vi "Signal Monitor.vi"() -> ()   [LabVIEW 2010]
uses:
  DAQ configuration/port to indices.vi
  DataServer/command.ctl
  DataServer/command cluster.ctl
  support/method.ctl
  DAQ configuration/channel identifier.ctl
  DAQ configuration/Sensor array.ctl
panel:
  in  "Sensor Array":T1
  out "digital display":sgl[](array[numeric]) format="%.4e"
  out "scans acquired":u32
  in  "Chart":bool
  out "seconds":u32
  out "backlog":u32
  out "data server address":string="calcium"
  in  "Data Servers":string[](array[string])=["dataserver.cee.cornell.edu", "calcium.cee.cornell.edu"]
  in  "method":T3={"sampling interval"=0.1, "samples to average"=1, "data interval"=0.0, "stream data"=FALSE, "file path"=refnum, "command"={"command"=enum."Idle", "start time (ms)"=0, "Channel Indices"=[], "Scans per Sample"=1}} {"command"."Scans per Sample" min=1; "data interval" format="%.2f"; "samples to average" min=1 step=1; "sampling interval" format="%.2f"}
  in  "Data log status":bool
  in  "Enable Logging data":bool
  in  "colors":u32[](array[colorbox])=[16711680, 16770090, 6487897, 16777215, 16753241, 16738047, 52479, 2556143, 16711680, 16770090, 7470980, 16777215, 16753241, 16738047, 52479, 2556143]
  out "error":errorcluster
  out "chart":sgl[][](graph)
  in  "port":u16=6341
  out "connection ID":refnum<k5>
  out "quit":bool=TRUE
  in  "State":T6
  in  "Stop":bool
  in  "Log Data":bool
  out "logging data to file:":path=path "C:/WINNT/Profiles/mlws/Desktop/50Hzjunk"
  # "current value"
  # "channel  name (units)"
  # "s"
  # "s"
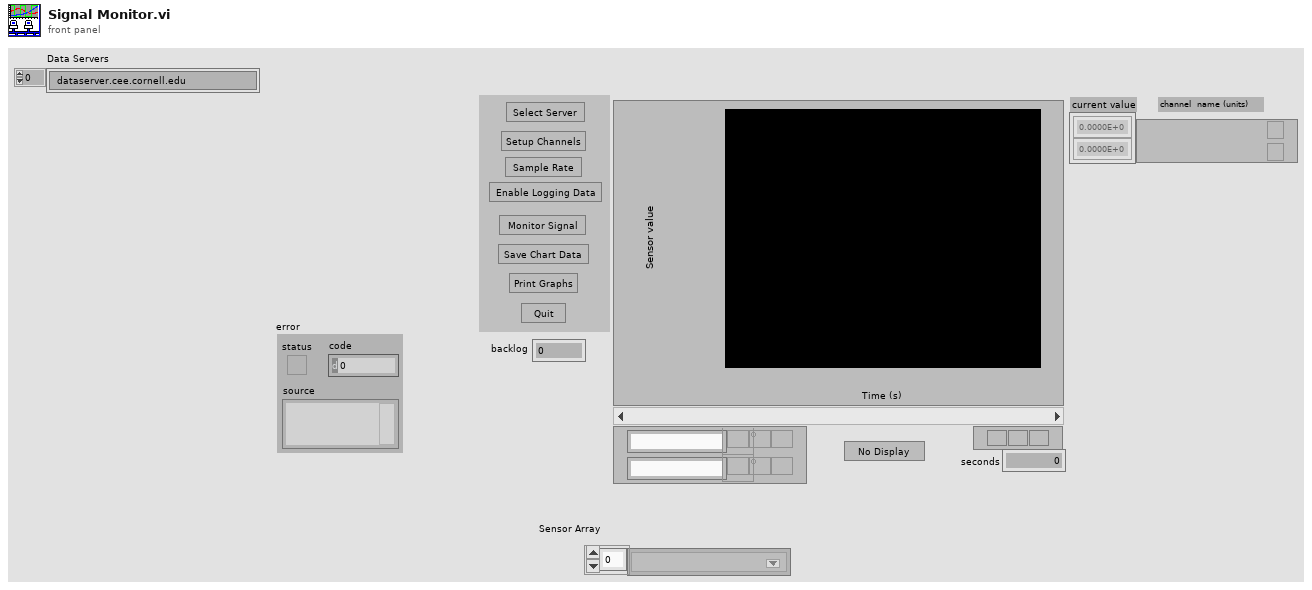
[diagram p1: front panel]
types:
  T1 = typedef "Sensor array.ctl" = T2[]
  T2 = typedef "channel identifier.ctl" = u16
  T3 = typedef "method.ctl" = cluster{"sampling interval":sgl, "samples to average":u32, "data interval":sgl, "stream data":bool, "file path":refnum<file>, "command":T4}
  T4 = typedef "command cluster.ctl" = cluster{"command":T5, "start time (ms)":u32, "Channel Indices":i32[], "Scans per Sample":i32}
  T5 = typedef "command.ctl" = enum16{"Idle", "Send Data", "Send 1 Scan", "Logoff"}
  T6 = cluster{"Quit":bool, "Select Server":bool, "Calibration":bool, "Set Rate":bool, "Monitor sample":bool, "Save data":bool, "Print graphs":bool}
  T7 = enum16{"Idle", "Send Data", "Send 1 Scan", "Logoff"}
  T8 = typedef "Sensor array.ctl" = T9[]
  T9 = typedef "sensor configuration.ctl" = cluster{"Port":T10, "calibration type":T11, "name":string}
  T10 = typedef "channel identifier.ctl" = cluster{"module":u8, "channel":u8}
  T11 = typedef "calibration type.ctl" = enum16{"None (raw voltage)", "From File", "Zero voltage", "Set calibrated output", "pH", "Dissolved Oxygen", "LVDT calibrator", "NF90 calibrator"}
  T12 = cluster{"X Scale Fit":u8, "Xo and delta X":cluster{"Xo":dbl, "delta X":dbl}, "X style":u8, "X Format & Precision":cluster{"X Format":u8, "X Precision":u8}, "X Range":cluster{"X Minimum":dbl, "X Maximum":dbl, "X Increment":dbl}, "X Flipped":bool, "X Mapping Mode":u8, "X Editable":bool}
  T13 = cluster{"Y Scale Fit":u8, "Yo and delta Y":cluster{"Yo":dbl, "delta Y":dbl}, "Y Style":u8, "Y Format & Precision":cluster{"Y Format":u8, "Y Precision":u8}, "Y Range":cluster{"Y Minimum":dbl, "Y Maximum":dbl, "Y Increment":dbl}, "Y Flipped":bool, "Y Mapping Mode":u8, "Y Editable":bool}
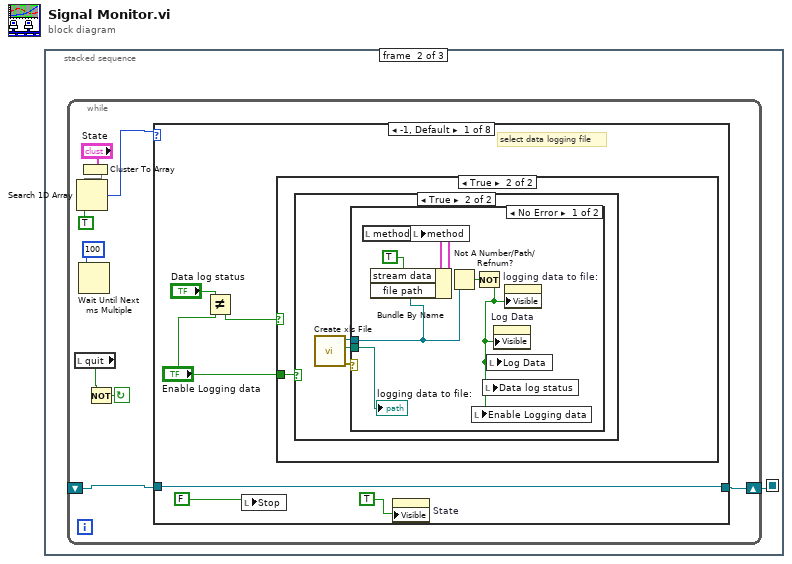
[diagram p0: block diagram]
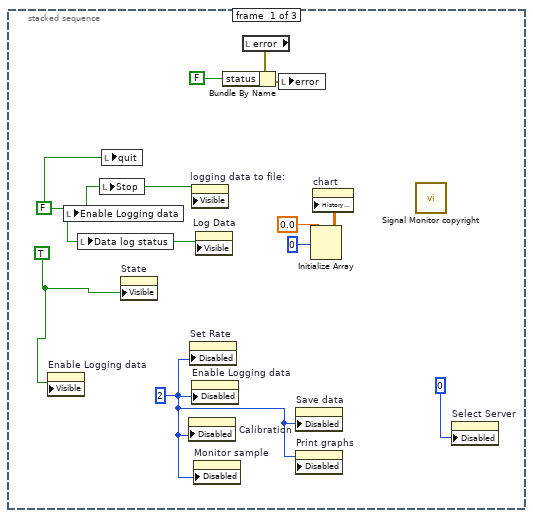
[diagram p2: hidden frame]
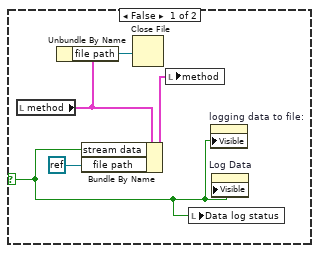
[diagram p4: hidden frame]
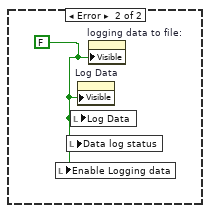
[diagram p5: hidden frame]
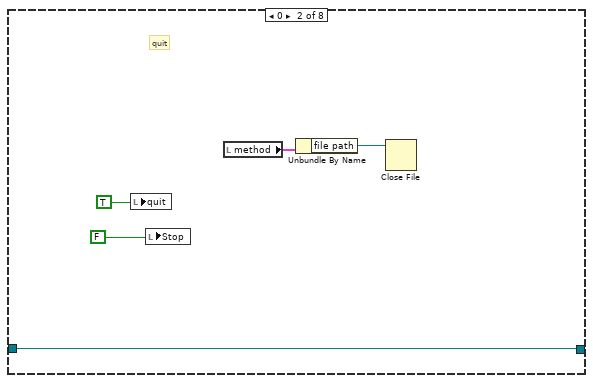
[diagram p6: hidden frame]
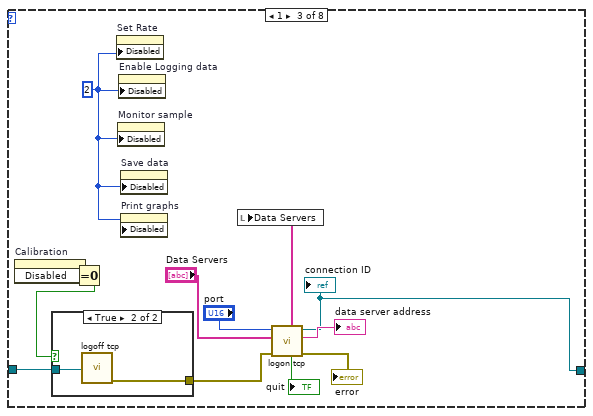
[diagram p7: hidden frame]
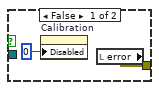
[diagram p8: hidden frame]
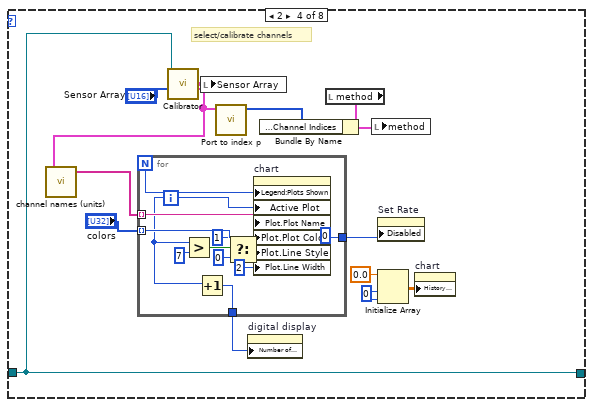
[diagram p9: hidden frame]
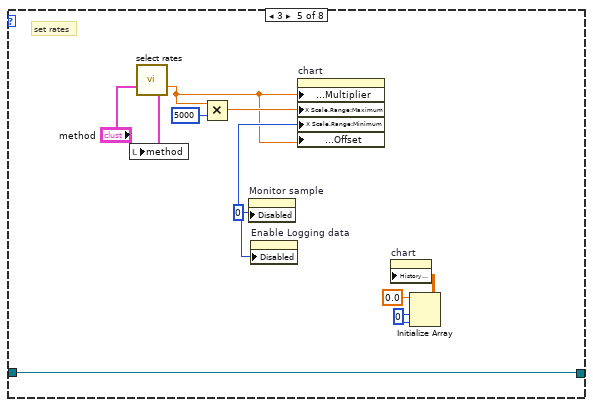
[diagram p10: hidden frame]
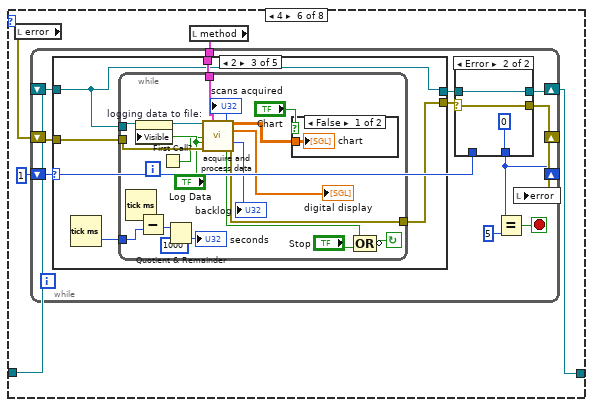
[diagram p11: hidden frame]
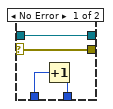
[diagram p12: hidden frame]
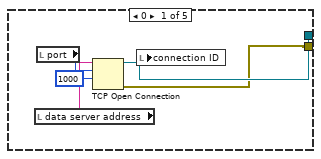
[diagram p13: hidden frame]
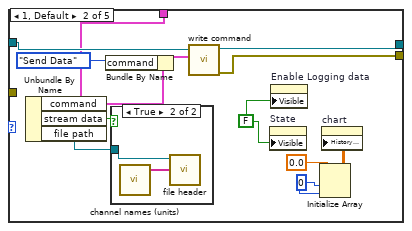
[diagram p14: hidden frame]
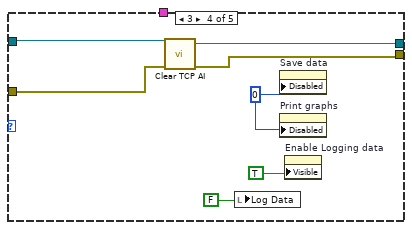
[diagram p17: hidden frame]
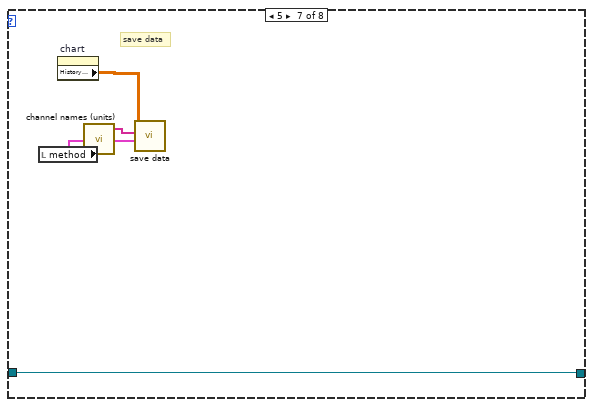
[diagram p19: hidden frame]
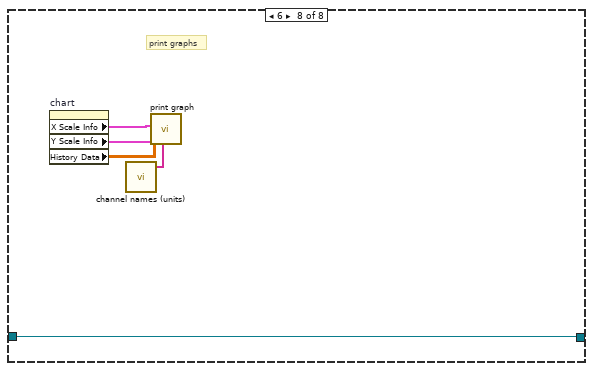
[diagram p20: hidden frame]
diagram:
  n1 = stacked-sequence {
    seq-local: [_ w11 _] -> [_ _ w186]
    frame #0 {
      w6 = TRUE
      w5 = 2
      w8 = 0
      w7 = FALSE
      n2 = property on="Enable Logging data" class="Bool (strict)"("Visible"=w6) -> ()  [unwired: 2 in, 2 out]
      n3 = local write "Enable Logging data"(w7) -> ()
      n4 = local write "Data log status"(w7) -> ()
      n5 = local write "Stop"(w7) -> ()
      n6 = local write "quit"(w7) -> ()
      n7 = property on="State" class="Clust"("Visible"=w6) -> ()  [unwired: 2 in, 2 out]
      n8 = property on="Calibration" class="Bool"("Disabled"=w5) -> ()  [unwired: 2 in, 2 out]
      n9 = property on="Set Rate" class="Bool"("Disabled"=w5) -> ()  [unwired: 2 in, 2 out]
      n10 = property on="logging data to file:" class="Path"("Visible"=w7) -> ()  [unwired: 2 in, 2 out]
      n11 = property on="Enable Logging data" class="Bool (strict)"("Disabled"=w5) -> ()  [unwired: 2 in, 2 out]
      n12 = property on="Monitor sample" class="Bool"("Disabled"=w5) -> ()  [unwired: 2 in, 2 out]
      n13 = property on="Log Data" class="Bool (strict)"("Visible"=w7) -> ()  [unwired: 2 in, 2 out]
      n14 = local read "error"() -> (w3:errorcluster)
      n15 = Bundle By Name(cluster=w3, "status"=FALSE ("Bundle Element")) -> (w2:errorcluster)
      n16 = local write "error"(w2) -> ()
      n17 = property on="Save data" class="Bool"("Disabled"=w5) -> ()  [unwired: 2 in, 2 out]
      n18 = property on="Print graphs" class="Bool"("Disabled"=w5) -> ()  [unwired: 2 in, 2 out]
      n19 = Initialize Array(sgl 0.0, w8, w8) -> (w9:sgl[][])
      n20 = property on="chart" class="WFChart (strict)"("History Data"=w9) -> ()  [unwired: 2 in, 2 out]
      n21 = call "Signal Monitor copyright"() -> ()  [unwired: 8 in]
      n22 = property on="Select Server" class="Bool"("Disabled"=u8 0 ("Write Attribute")) -> ()  [unwired: 2 in, 2 out]
    }
    frame #1 {
      n23 = while {
        shift-left: _ -> [w13]
        shift-right: [w12] -> w11
        stop <- w19 continue-if-true
        n24 = local read "quit"() -> (w20:bool)
        n25 = Wait Until Next ms Multiple(millisecond multiple=100) -> ()  [unwired: 1 out]
        n26 = Cluster To Array(cluster="State") -> (array=w17:bool[])
        n27 = Search 1D Array(1D array=w17, element=TRUE) -> (index of element=w16:i32)  [unwired: 1 in]
        n28 = Not(x=w20) -> (.not. x?=w19:bool)
        n29 = case shown="-1, Default" w16 {
          tunnel: w13 -> [w21 w46 w54 w77 w94 w103 w177 w181]
          tunnel: [w21 w46 w56 w77 w94 w102 w177 w181] -> w12
          frame -1, Default {
            # "select data logging file"
            n30 = Not Equal?(x="Data log status", y="Enable Logging data") -> (x != y?=w22:bool)
            n31 = local write "Stop"(FALSE) -> ()
            n32 = case shown="True" w22 {
              tunnel: "Enable Logging data" -> [_ w27]
              frame False {
              }
              frame True {
                n33 = case shown="True" w27 {
                  selector: w27 -> [w30 _]
                  frame False {
                    n34 = local read "method"() -> (w29:T3)
                    n35 = Unbundle By Name(w29) -> ("file path"=w28:refnum<file>)
                    n36 = Bundle By Name(cluster=w29, "stream data"=w30, "file path"=refnum<k0> refnum) -> (w32:T3)
                    n37 = Close File(refnum=w28) -> ()  [unwired: 1 in, 2 out]
                    n38 = local write "method"(w32) -> ()
                    n39 = local write "Data log status"(w30) -> ()
                    n40 = property on="logging data to file:" class="Path"("Visible"=w30) -> ()  [unwired: 2 in, 2 out]
                    n41 = property on="Log Data" class="Bool (strict)"("Visible"=w30) -> ()  [unwired: 2 in, 2 out]
                  }
                  frame True {
                    n42 = call "Create xls File.vi"() -> ("error out"=w34:errorcluster, "path"=w33:path, "refnum"=w35:refnum<file>)  [unwired: 4 in, 1 out]
                    n43 = case shown="No Error" w34 {
                      tunnel: w35 -> [w36 _]
                      tunnel: w33 -> [w37 _]
                      frame No Error {
                        n44 = local read "method"() -> (w40:T3)
                        n45 = Bundle By Name(cluster=w40, "stream data"=TRUE, "file path"=w36) -> (w41:T3)
                        n46 = local write "method"(w41) -> ()
                        n47 = Not A Number/Path/Refnum?(number/path/refnum=w36) -> (NaN/Path/Refnum?=w38:bool)
                        n48 = Not(x=w38) -> (.not. x?=w39:bool)
                        n49 = local write "Enable Logging data"(w39) -> ()
                        n50 = local write "Data log status"(w39) -> ()
                        n51 = local write "Log Data"(w39) -> ()
                        n52 = property on="Log Data" class="Bool (strict)"("Visible"=w39) -> ()  [unwired: 2 in, 2 out]
                        n53 = property on="logging data to file:" class="Path"("Visible"=w39) -> ()  [unwired: 2 in, 2 out]
                        "logging data to file:" <- w37
                      }
                      frame Error {
                        w43 = FALSE
                        n54 = local write "Enable Logging data"(w43) -> ()
                        n55 = local write "Data log status"(w43) -> ()
                        n56 = local write "Log Data"(w43) -> ()
                        n57 = property on="Log Data" class="Bool (strict)"("Visible"=w43) -> ()  [unwired: 2 in, 2 out]
                        n58 = property on="logging data to file:" class="Path"("Visible"=w43) -> ()  [unwired: 2 in, 2 out]
                      }
                    }
                  }
                }
              }
            }
            n59 = property on="State" class="Clust"("Visible"=TRUE) -> ()  [unwired: 2 in, 2 out]
          }
          frame 0 {
            # "quit"
            n60 = local write "quit"(TRUE) -> ()
            n61 = local write "Stop"(FALSE) -> ()
            n62 = local read "method"() -> (w45:T3)
            n63 = Unbundle By Name(w45) -> ("file path"=w44:refnum<file>)
            n64 = Close File(refnum=w44) -> ()  [unwired: 1 in, 2 out]
          }
          frame 1 {
            w53 = 2
            n65 = property on="Calibration" class="Bool"() -> ("Disabled"=w52:u8)  [unwired: 2 in, 2 out]
            n66 = Equal To 0?(x=w52) -> (x = 0?=w51:bool)
            n67 = case shown="True" w51 {
              tunnel: w54 -> [_ w64]
              tunnel: [w61 w63] -> w50
              frame False {
                n68 = property on="Calibration" class="Bool"("Disabled"=u8 0 ("Write Attribute")) -> ()  [unwired: 2 in, 2 out]
                n69 = local read "error"() -> (w61:errorcluster)
              }
              frame True {
                n70 = call "logoff tcp.vi"("Connection ID"=w64) -> ("error out"=w63:errorcluster)  [unwired: 9 in, 1 out]
              }
            }
            n71 = property on="Set Rate" class="Bool"("Disabled"=w53) -> ()  [unwired: 2 in, 2 out]
            n72 = property on="Monitor sample" class="Bool"("Disabled"=w53) -> ()  [unwired: 2 in, 2 out]
            n73 = property on="Enable Logging data" class="Bool (strict)"("Disabled"=w53) -> ()  [unwired: 2 in, 2 out]
            n74 = property on="Save data" class="Bool"("Disabled"=w53) -> ()  [unwired: 2 in, 2 out]
            n75 = property on="Print graphs" class="Bool"("Disabled"=w53) -> ()  [unwired: 2 in, 2 out]
            n76 = call "logon tcp.vi"("error in"=w50, "Data Servers"="Data Servers", "port"="port") -> ("error out"=→"error":errorcluster, "data server address"=→"data server address":string, "connection ID"=w56:refnum<k5>, "restart"=→"quit":bool, "Data Servers out"=w49:string[])  [unwired: 3 in, 1 out]
            "connection ID" <- w56
            n77 = local write "Data Servers"(w49) -> ()
          }
          frame 2 {
            w73 = 0
            # "select/calibrate channels"
            n78 = call "Calibrator.vi"("Sensor Array"="Sensor Array", "Connection ID"=w77) -> ("Sensor Array out"=w65:T8)  [unwired: 8 in, 1 out]
            n79 = call "channel names (units).vi"("Sensor Array"=w65) -> ("channel strings"=w76:string[])  [unwired: 4 in]
            n80 = for {
              N -> [w79]
              tunnel: w76 -> [w89] mode=indexing
              tunnel: "colors" -> [w88] mode=indexing
              tunnel: [0] -> w74
              tunnel: [w80] -> w75
              i -> [w81]
              n81 = Greater?(x=w81, y=7) -> (0:w87:bool)
              n82 = Increment(x=w81) -> (x+1=w80:i32)
              n83 = Select(t=1, s=w87, f=0) -> (s? t:f=w84:i32)
              n84 = property on="chart" class="WFChart (strict)"("Legend:Plots Shown"=w79, "Active Plot"=w81, "Plot.Plot Name"=w89, "Plot.Plot Color"=w88, "Plot.Line Style"=w84, "Plot.Line Width"=u8 2) -> ()  [unwired: 2 in, 2 out]
            }
            n85 = local write "Sensor Array"(w65) -> ()
            n86 = call-poly "Port to index p.vi"("Port"=w65) -> ("Channel Indices"=w69:i32[])  [unwired: 10 in]
            n87 = property on="digital display" class="Arr (strict)"("Number of Rows"=w75) -> ()  [unwired: 2 in, 2 out]
            n88 = local read "method"() -> (w67:T3)
            n89 = Bundle By Name(cluster=w67, "command.Channel Indices"=w69) -> (w68:T3)
            n90 = local write "method"(w68) -> ()
            n91 = property on="Set Rate" class="Bool"("Disabled"=w74) -> ()  [unwired: 2 in, 2 out]
            n92 = Initialize Array(sgl 0.0, w73, w73) -> (w71:sgl[][])
            n93 = property on="chart" class="WFChart (strict)"("History Data"=w71) -> ()  [unwired: 2 in, 2 out]
          }
          frame 3 {
            w95 = 0
            w92 = 0
            # "set rates"
            n94 = call "select rates.vi"("method in"="method") -> ("method out"=w93:T3, "new data interval"=w90:sgl)  [unwired: 10 in, 3 out]
            n95 = local write "method"(w93) -> ()
            n96 = Multiply(x=w90, y=5000) -> (x*y=w98:sgl)
            n97 = property on="Monitor sample" class="Bool"("Disabled"=w92) -> ()  [unwired: 2 in, 2 out]
            n98 = property on="Enable Logging data" class="Bool (strict)"("Disabled"=w92) -> ()  [unwired: 2 in, 2 out]
            n99 = property on="chart" class="WFChart (strict)"("X Scale.Offset and Multiplier:Multiplier"=w90, "X Scale.Range:Maximum"=w98, "X Scale.Range:Minimum"=w92, "X Scale.Offset and Multiplier:Offset"=w90) -> ()  [unwired: 2 in, 2 out]
            n100 = Initialize Array(sgl 0.0, w95, w95) -> (w97:sgl[][])
            n101 = property on="chart" class="WFChart (strict)"("History Data"=w97) -> ()  [unwired: 2 in, 2 out]
          }
          frame 4 {
            n102 = local read "error"() -> (w101:errorcluster)
            n103 = local read "method"() -> (w104:T3)
            n104 = while {
              shift-left: w103 -> [w113]
              shift-right: [w111] -> w102
              shift-left: 1 -> [w112]
              shift-right: [w108] -> _
              tunnel: w104 -> [w114]
              shift-left: w101 -> [w115]
              shift-right: [w109] -> _
              stop <- w106 stop-if-true
              n105 = case shown="2" w112 {
                tunnel: [w123 w139 w145 w170 _] -> w105
                tunnel: w115 -> [_ _ w147 w171 _]
                tunnel: w114 -> [_ w137 w146 _ _]
                tunnel: w113 -> [_ w138 w143 w169 w175]
                tunnel: [w124 w128 w143 w168 w175] -> w110
                frame 0 {
                  n106 = local read "data server address"() -> (w126:string)
                  n107 = local read "port"() -> (w125:u16)
                  n108 = TCP Open Connection(address=w126, remote port or service name=w125, timeout ms (60000)=1000) -> (connection ID=w124:refnum<k5>, error out=w123:errorcluster)  [unwired: 2 in]
                  n109 = local write "connection ID"(w124) -> ()
                }
                frame 1, Default {
                  w132 = 0
                  w133 = FALSE
                  n110 = Unbundle By Name(w137) -> ("command"=w134:T4, "stream data"=w135:bool, "file path"=w136:refnum<file>)
                  n111 = Bundle By Name(cluster=w134, "command"=T7."Send Data") -> (w140:T4)
                  n112 = case shown="True" w135 {
                    tunnel: w136 -> [_ w142]
                    frame False {
                    }
                    frame True {
                      n113 = call "channel names (units).vi"() -> ("channel strings"=w141:string[])  [unwired: 5 in]
                      n114 = call "file header.vi"("channel strings"=w141, "refnum"=w142) -> ()  [unwired: 9 in, 1 out]
                    }
                  }
                  n115 = call "write command.vi"("command interface"=w140, "refnum in"=w138) -> ("error out"=w139:errorcluster, "refnum out"=w128:refnum<k5>)  [unwired: 8 in]
                  n116 = property on="State" class="Clust"("Visible"=w133) -> ()  [unwired: 2 in, 2 out]
                  n117 = property on="Enable Logging data" class="Bool (strict)"("Visible"=w133) -> ()  [unwired: 2 in, 2 out]
                  n118 = Initialize Array(sgl 0.0, w132, w132) -> (w130:sgl[][])
                  n119 = property on="chart" class="WFChart (strict)"("History Data"=w130) -> ()  [unwired: 2 in, 2 out]
                }
                frame 2 {
                  n120 = Tick Count (ms)() -> (millisecond timer value=w144:u32)
                  n121 = while {
                    tunnel: w144 -> [w156]
                    tunnel: w143 -> [w157]
                    tunnel: w146 -> [w158]
                    tunnel: [w162] -> w145
                    tunnel: w147 -> [w161]
                    stop <- w166 continue-if-true
                    n122 = Tick Count (ms)() -> (millisecond timer value=w155:u32)
                    n123 = property on="logging data to file:" class="Path"("Visible"="Log Data") -> ()  [unwired: 2 in, 2 out]
                    n124 = Subtract(x=w155, y=w156) -> (x-y=w153:u32)
                    n125 = First Call?() -> (First Call?: T/F=w148:bool)
                    n126 = Quotient & Remainder(x=w153, y=u32 1000) -> (floor(x/y)=→"seconds":u32)  [unwired: 1 out]
                    n127 = call "acquire and process data.vi"("connection ID"=w157, "Reset"=w148, "Log Data"="Log Data", "error in"=w161, "method"=w158) -> ("samples"=→"scans acquired":u32, "data out"=w164:sgl[][], "last reading"=→"digital display":sgl[], "backlog"=→"backlog":u32, "Status"=w159:bool, "error out"=w162:errorcluster)  [unwired: 3 in, 2 out]
                    n128 = case shown="False" "Chart" {
                      tunnel: w164 -> [w167 _]
                      frame False {
                        "chart" <- w167
                      }
                      frame True {
                      }
                    }
                    n129 = Compound Arithmetic op=OR(w159, "Stop") -> (invert w166:bool)
                  }
                }
                frame 3 {
                  w173 = 0
                  n130 = call "Clear TCP AI.vi"("error in (no error)"=w171, "Connection ID in"=w169) -> ("error out"=w170:errorcluster, "Connection ID out"=w168:refnum<k5>)  [unwired: 8 in]
                  n131 = local write "Log Data"(FALSE) -> ()
                  n132 = property on="Save data" class="Bool"("Disabled"=w173) -> ()  [unwired: 2 in, 2 out]
                  n133 = property on="Print graphs" class="Bool"("Disabled"=w173) -> ()  [unwired: 2 in, 2 out]
                  n134 = property on="Enable Logging data" class="Bool (strict)"("Visible"=TRUE) -> ()  [unwired: 2 in, 2 out]
                }
                frame 4 {
                  # "stop"
                }
              }
              n135 = case shown="Error" w105 {
                selector: w105 -> [w116 w120]
                tunnel: w112 -> [w119 _]
                tunnel: [w118 0] -> w108
                tunnel: [w117 w121] -> w111
                tunnel: w110 -> [w117 w121]
                tunnel: [w116 w120] -> w109
                frame No Error {
                  n136 = Increment(x=w119) -> (x+1=w118:i32)
                }
                frame Error {
                }
              }
              n137 = Equal?(x=w108, y=5) -> (x = y?=w106:bool)
              n138 = local write "error"(w109) -> ()
            }
          }
          frame 5 {
            # "save data"
            n139 = local read "method"() -> (w179:T3)
            n140 = property on="chart" class="WFChart (strict)"() -> ("History Data"=w178:sgl[][])  [unwired: 2 in, 2 out]
            n141 = call "channel names (units).vi"() -> ("channel strings"=w176:string[])  [unwired: 5 in]
            n142 = call "save data.vi"("method"=w179, "channel strings"=w176, "voltage data"=w178) -> ()  [unwired: 9 in]
          }
          frame 6 {
            # "print graphs"
            n143 = property on="chart" class="WFChart (strict)"() -> ("X Scale Info"=w184:T12, "Y Scale Info"=w183:T13, "History Data"=w182:sgl[][])  [unwired: 2 in, 2 out]
            n144 = call "channel names (units).vi"() -> ("channel strings"=w180:string[])  [unwired: 5 in]
            n145 = call "print graph.vi"("channel strings"=w180, "History Data"=w182, "Y Scale Info"=w183, "X Scale Info"=w184) -> ()  [unwired: 8 in]
          }
        }
      }
    }
    frame #2 {
      n146 = local read "error"() -> (w185:errorcluster)
      n147 = case shown="No Error" w185 {
        selector: w185 -> [_ w199]
        tunnel: w186 -> [w192 _]
        frame No Error {
          n148 = property on="Calibration" class="Bool"() -> ("Disabled"=w191:u8)  [unwired: 2 in, 2 out]
          n149 = Equal To 0?(x=w191) -> (x = 0?=w190:bool)
          n150 = case shown="False" w190 {
            tunnel: w192 -> [_ w195]
            tunnel: [FALSE ("Front Panel Window:Open") FALSE ("Front Panel Window:Open")] -> w187
            frame False {
            }
            frame True {
              n151 = call "logoff tcp.vi"("Connection ID"=w195) -> ()  [unwired: 9 in, 2 out]
            }
          }
          n152 = property class="VI"("Front Panel Window:Open"=w187) -> (reference out=w189:refnum<vi>, error out=w188:errorcluster)  [unwired: 2 in]
          n153 = Close Reference(reference=w189, error in (no error)=w188) -> ()  [unwired: 1 out]
        }
        frame Error {
          n154 = Unbundle By Name(w199) -> ("status"=w196:bool)
          n155 = property on="State" class="Clust"("Visible"=w196) -> ()  [unwired: 2 in, 2 out]
          n156 = local write "Stop"(FALSE) -> ()
          n157 = One Button Dialog(message="Connection with the data server was lost. Signal Monitor was disconnected from the Data Server. Restart this program and use a lower data rate or turn off the graph updates.") -> ()  [unwired: 1 in, 1 out]
        }
      }
    }
  }
